vi "18_AcquisitionDataProgram.vi"() -> ()   [LabVIEW 2015]
uses:
  <vilib>/Analysis/4window.llb/windowTd.ctl
  <vilib>/DAQmx/configure/timing.llb/DAQmx Timing (Sample Clock).vi
  <vilib>/DAQmx/miscellaneous.llb/DAQmx Fill In Error Info.vi
  <vilib>/measure/maspectr.llb/FFT Power Spectrum and PSD for 1 Chan.vi
  <vilib>/DAQmx/create/channels.llb/DAQmx Create Channel (AO-Voltage-Basic).vi
  <vilib>/DAQmx/create/channels.llb/DAQmx Create Channel (AI-Voltage-Basic).vi
  <vilib>/DAQmx/read.llb/DAQmx Read (Analog Wfm 1Chan NSamp).vi
  <vilib>/measure/matone.llb/Extract Single Tone Information 1 Chan.vi
  <vilib>/DAQmx/write.llb/DAQmx Write (Analog Wfm 1Chan NSamp).vi
  <vilib>/Utility/file.llb/Write Delimited Spreadsheet (string).vi
  <vilib>/measure/NI_MABase.lvlib
  <vilib>/measure/NI_MAPro.lvlib
  <vilib>/Analysis/NI_AALPro.lvlib
panel:
  in  "Tab Control":enum32{"Page 1", "Page 2"}(tab)
  out "Waveform Graph 3":cluster{"f0":dbl, "df":dbl, "magnitude":dbl[]}(graph)
  out "Waveform Graph 2":waveform(dbl)(graph)
  out "detected frequency":dbl format="%.2p"
  out "Boolean":bool
  out "Boolean 2":bool
  out "Boolean 3":bool
  out "Boolean 4":bool
  out "Boolean 5":bool
  out "Boolean 6":bool
  in  "Save Button":bool
  in  "file path (dialog if empty)":path=path "C:/Users/student/Desktop/GrellaMarsellaOliva/configuration_tree.txt.txt"
  in  "physical channels 2":tag="Dev1/ai2"
  in  "window":T1=1 items=["Rectangle"=0, "Hanning"=1, "Hamming"=2, "Blackman-Harris"=3, "Exact Blackman"=4, "Blackman"=5, "Flat Top"=6, "4 Term B-Harris "=7, "7 Term B-Harris"=8, "Low Sidelobe"=9, "Blackman Nuttall"=11, "Triangle"=30, "Bartlett-Hanning"=31, "Bohman"=32, "Parzen"=33, "Welch"=34, "Kaiser"=60, "Dolph-Chebyshev"=61, "Gaussian"=62]
  in  "dB On":bool
  out "detected amplitude":dbl format="%.2p"
  out "Waveform Graph":waveform(dbl)(graph)
  in  "rate":string(combo)="20"
  in  "physical channels":tag="Dev1/ao0"
  in  "amplitude":dbl(knob)=2.0 scale=0.0..5.0
  in  "stop":bool
  # "Luca Grellla, Daniele Marsella, Gianluigi Oliva"
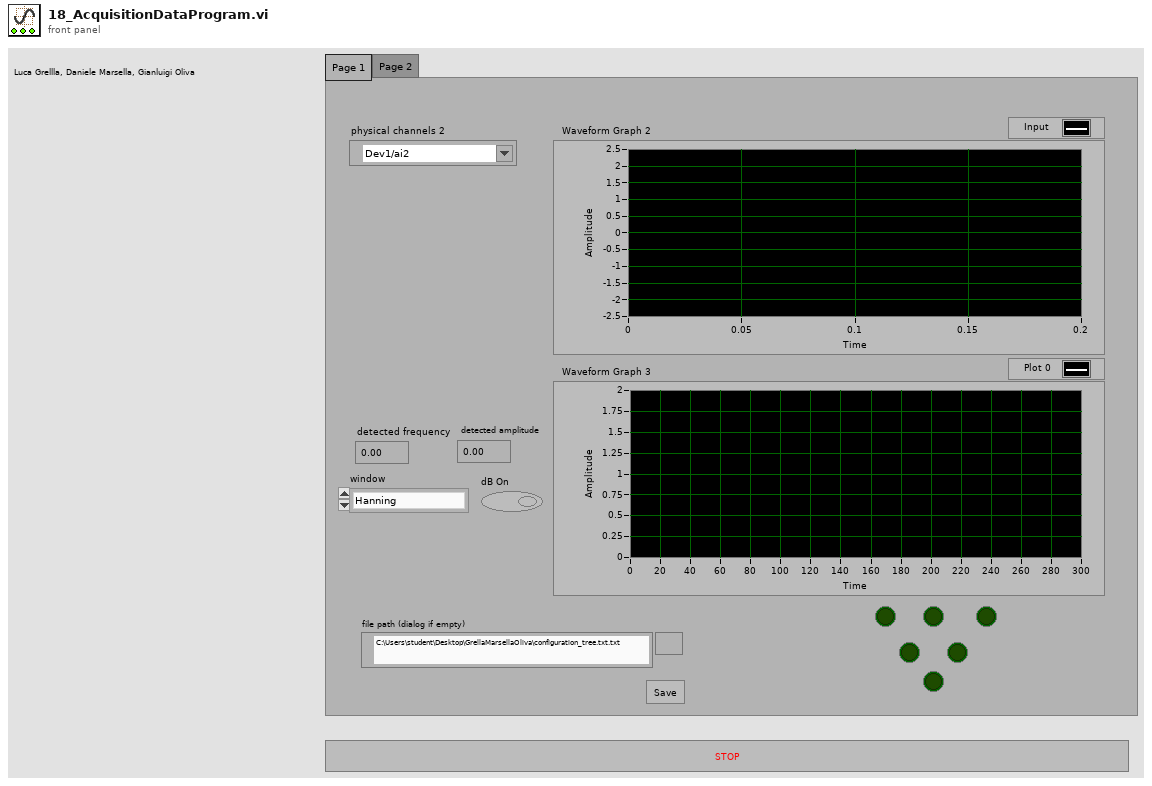
[diagram p1: front panel]
types:
  T1 = typedef "NI_AALPro.lvlib/windowTd.ctl" = u32
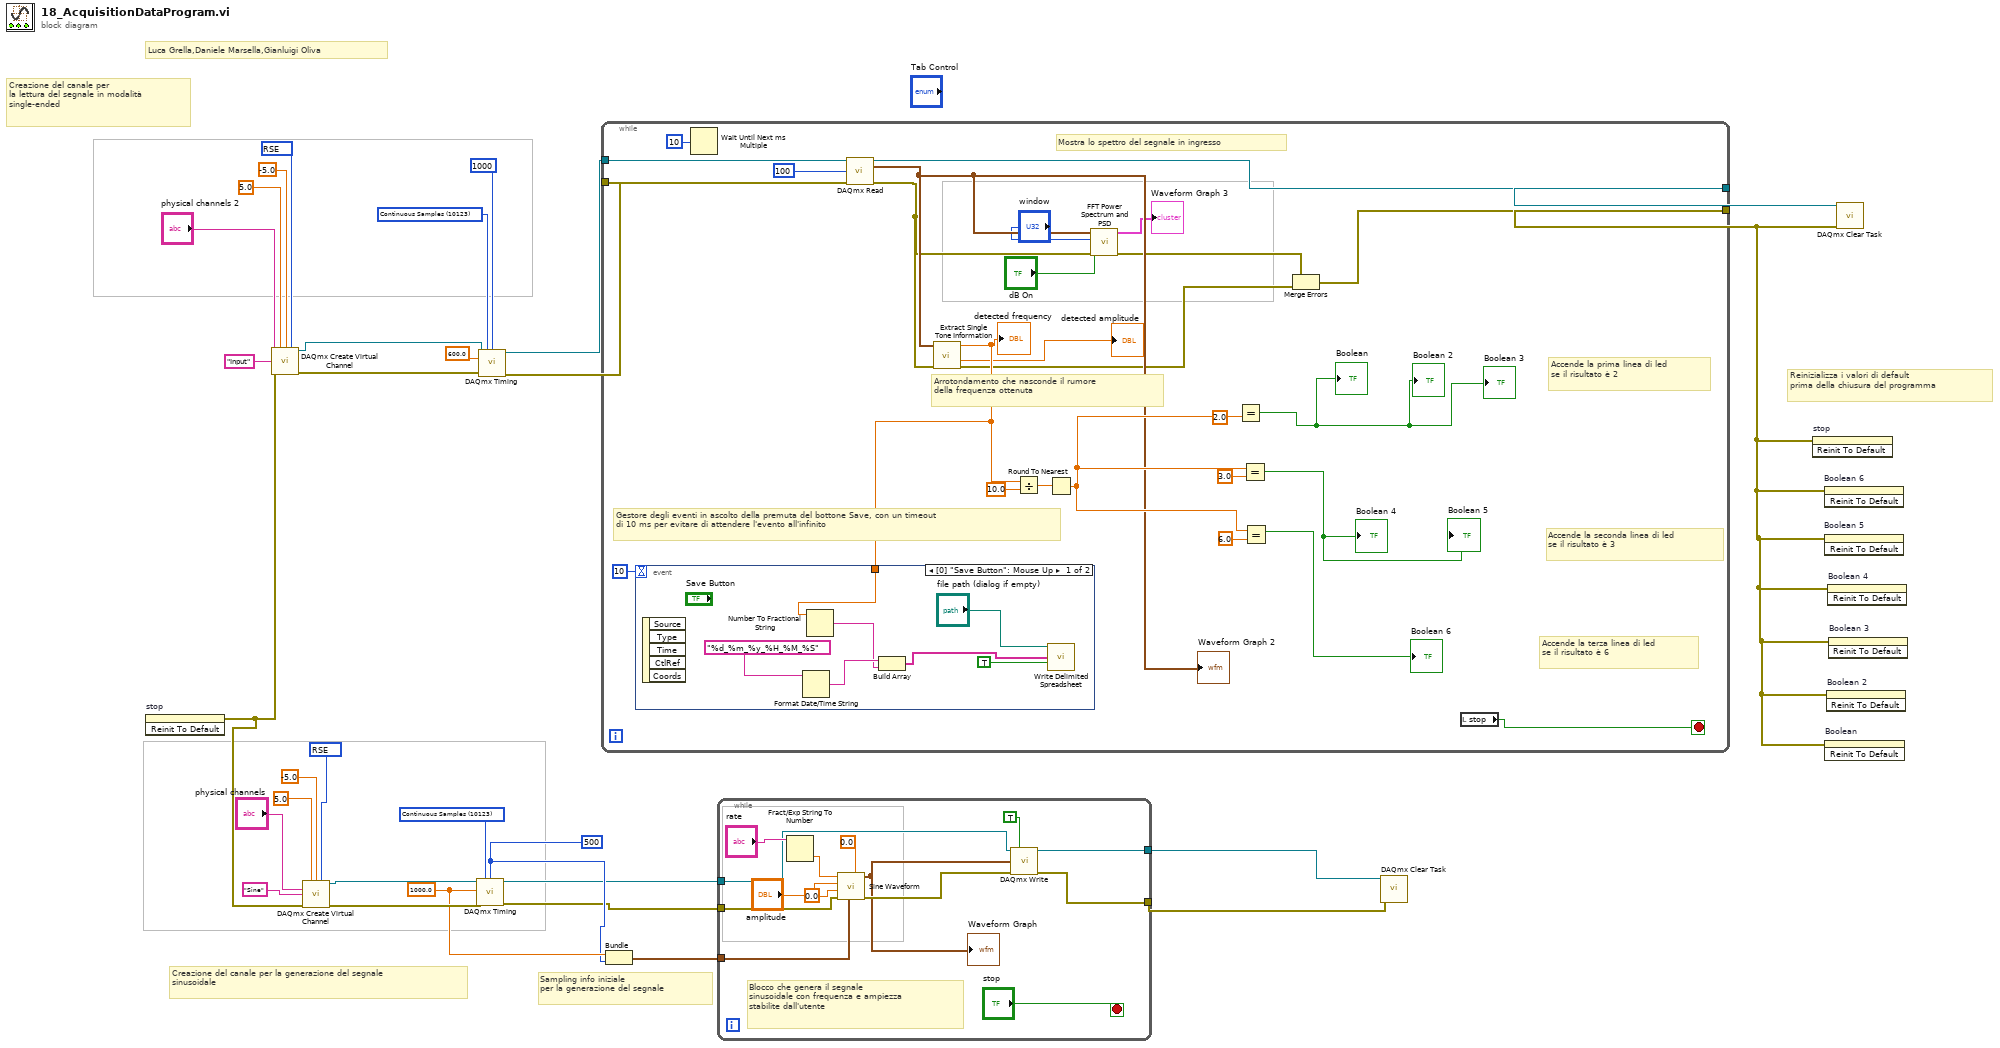
[diagram p0: block diagram]
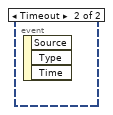
[diagram p2: hidden frame]
diagram:
  w3 = 10083 items=["Default"=-1, "RSE"=10083, "NRSE"=10078, "Differential"=10106, "Pseudodifferential"=12529] ("input terminal configuration")
  w12 = 10123 items=["Finite Samples"=10178, "Continuous Samples"=10123, "Hardware Timed Single Point"=12522] ("sample mode")
  w21 = 500 ("samples per channel")
  w22 = 1000.0 ("rate")
  w24 = 10123 items=["Finite Samples"=10178, "Continuous Samples"=10123, "Hardware Timed Single Point"=12522] ("sample mode")
  w27 = 10083 items=["Default"=-1, "RSE"=10083, "Differential"=10106, "Pseudodifferential"=12529] ("output terminal configuration")
  # "Reinizializza i valori di default\nprima della chiusura del programma"
  # "Sampling info iniziale\nper la generazione del segnale"
  # "Creazione del canale per la generazione del segnale \nsinusoidale"
  # "Creazione del canale per\nla lettura del segnale in modalità\nsingle-ended"
  # "Luca Grella,Daniele Marsella,Gianluigi Oliva"
  n1 = invoke on="stop" class="Bool (strict)" method="Reinit To Default"() -> (error out=w6:errorcluster)  [unwired: 3 in, 2 out]
  n2 = call-poly <vilib>:"DAQmx Create Virtual Channel.vi"("maximum value"=5.0, "minimum value"=-5.0, "input terminal configuration"=w3, "physical channels"="physical channels 2", "name to assign"="Input", "error in"=w6) -> ("task out"=w11:refnum<k21>, "error out"=w10:errorcluster)  [unwired: 8 in]
  n3 = call-poly <vilib>:"DAQmx Create Virtual Channel.vi"("maximum value"=5.0, "minimum value"=-5.0, "output terminal configuration"=w27, "physical channels"="physical channels", "name to assign"="Sine", "error in"=w6) -> ("task out"=w25:refnum<k21>, "error out"=w23:errorcluster)  [unwired: 8 in]
  n4 = call-poly <vilib>:"DAQmx Timing.vi"("task/channels in"=w25, "sample mode"=w24, "samples per channel"=w21, "rate"=w22, "error in"=w23) -> ("task out"=w19:refnum<k21>, "error out"=w18:errorcluster)  [unwired: 9 in]
  n5 = call-poly <vilib>:"DAQmx Timing.vi"("task/channels in"=w11, "sample mode"=w12, "samples per channel"=1000, "rate"=600.0, "error in"=w10) -> ("task out"=w8:refnum<k21>, "error out"=w7:errorcluster)  [unwired: 9 in]
  n6 = while {
    tunnel: w8 -> [w56]
    tunnel: w7 -> [w55]
    tunnel: [w53] -> w2
    tunnel: [w33] -> w1
    stop <- w54 stop-if-true
    # "Mostra lo spettro del segnale in ingresso"
    # "Accende la terza linea di led\nse il risultato è 6"
    # "Accende la seconda linea di led\nse il risultato è 3"
    # "Accende la prima linea di led\nse il risultato è 2"
    # "Arrotondamento che nasconde il rumore\ndella frequenza ottenuta"
    # "Gestore degli eventi in ascolto della premuta del bottone Save, con un timeout\ndi 10 ms per evitare di attendere l'evento all'infinito"
    n7 = Wait Until Next ms Multiple(millisecond multiple=u32 10) -> ()  [unwired: 1 out]
    n8 = call-poly <vilib>:"DAQmx Read.vi"("task/channels in"=w56, "number of samples per channel"=100 ("samples per channel"), "error in"=w55) -> ("task out"=w53:refnum<k21>, "data"=w39:waveform(dbl), "error out"=w36:errorcluster)  [unwired: 10 in]
    "Waveform Graph 2" <- w39
    n9 = call-poly <vilib>:"Extract Single Tone Information.vi"("error in (no error)"=w36, "time signal in"=w39) -> ("error out"=w35:errorcluster, "detected amplitude"=→"detected amplitude":dbl, "detected frequency"=w49:dbl)  [unwired: 4 in, 3 out]
    "detected frequency" <- w49
    n10 = event shown="[0] \"Save Button\": Mouse Up" {
      selector: _ -> [_ _]
      dyn-events: _ -> [_ _]
      timeout: 10 -> [_ _]
      tunnel: w49 -> [w59 _]
      event "Save Button": Mouse Up {
        n11 = event-data() -> ()  [unwired: 1 in, 5 out]
        n12 = Format Date/Time String(time format string (%c)="%d_%m_%y_%H_%M_%S") -> (date/time string=w62:string)  [unwired: 2 in]
        n13 = Number To Fractional String(number=w59) -> (F-format string=w58:string)  [unwired: 3 in]
        n14 = Build Array(w62, w58) -> (w57:string[])
        n15 = call-poly <vilib>:"Write Delimited Spreadsheet.vi"("file path (dialog if empty)"="file path (dialog if empty)", "1D data"=w57, "append to file? (F)"=TRUE) -> ()  [unwired: 11 in, 2 out]
      }
      event Timeout {
        n16 = event-data() -> ()  [unwired: 1 in, 3 out]
      }
    }
    n17 = Divide(x=w49, y=10.0) -> (x/y=w47:dbl)
    n18 = Round To Nearest(number=w47) -> (nearest integer value=w46:dbl)
    n19 = call-poly <vilib>:"FFT Power Spectrum and PSD.vi"("error in (no error)"=w36, "dB On (F)"="dB On", "window"="window", "time signal"=w39) -> ("error out"=w34:errorcluster, "Power Spectrum / PSD"=→"Waveform Graph 3":cluster{"f0":dbl, "df":dbl, "magnitude":dbl[]})  [unwired: 4 in, 2 out]
    n20 = Equal?(x=w46, y=2.0) -> (x = y?=→"Boolean" →"Boolean 2" →"Boolean 3":bool)
    n21 = Equal?(x=w46, y=3.0) -> (x = y?=→"Boolean 4" →"Boolean 5":bool)
    n22 = Equal?(x=w46, y=6.0) -> (x = y?=→"Boolean 6":bool)
    n23 = Merge Errors(w34, w35) -> (w33:errorcluster)
    n24 = local read "stop"() -> (w54:bool)
  }
  n25 = Bundle("rate"=w22, "samples per channel"=w21) -> (w20:cluster{"rate":dbl, "samples per channel":i32})  [unwired: 1 in]
  n26 = while {
    tunnel: w20 -> [w72]
    tunnel: w19 -> [w71]
    tunnel: w18 -> [w66]
    tunnel: [w70] -> w17
    tunnel: [w69] -> w16
    stop <- "stop" stop-if-true
    # "Blocco che genera il segnale \nsinusoidale con frequenza e ampiezza\nstabilite dall'utente"
    n27 = Fract/Exp String To Number(string="rate") -> (number=w76:dbl)  [unwired: 3 in, 1 out]
    n28 = call <vilib>:"Sine Waveform.vi"("offset"=0.0, "sampling info"=w72, "error in (no error)"=w66, "phase"=0.0, "amplitude"="amplitude", "frequency"=w76) -> ("error out"=w65:errorcluster, "signal out"=w64:waveform(dbl))  [unwired: 4 in]
    "Waveform Graph" <- w64
    n29 = call-poly <vilib>:"DAQmx Write.vi"("task/channels in"=w71, "auto start"=TRUE, "data"=w64, "error in"=w65) -> ("task out"=w70:refnum<k21>, "error out"=w69:errorcluster)  [unwired: 9 in, 1 out]
  }
  n30 = call <vilib>:"DAQmx Clear Task.vi"("task in"=w17, "error in"=w16) -> ()  [unwired: 13 in, 1 out]
  n31 = invoke on="stop" class="Bool (strict)" method="Reinit To Default"(error in=w1) -> ()  [unwired: 2 in, 3 out]
  n32 = invoke on="Boolean 6" class="Bool (strict)" method="Reinit To Default"(error in=w1) -> ()  [unwired: 2 in, 3 out]
  n33 = invoke on="Boolean 5" class="Bool (strict)" method="Reinit To Default"(error in=w1) -> ()  [unwired: 2 in, 3 out]
  n34 = invoke on="Boolean" class="Bool (strict)" method="Reinit To Default"(error in=w1) -> ()  [unwired: 2 in, 3 out]
  n35 = invoke on="Boolean 2" class="Bool (strict)" method="Reinit To Default"(error in=w1) -> ()  [unwired: 2 in, 3 out]
  n36 = invoke on="Boolean 4" class="Bool (strict)" method="Reinit To Default"(error in=w1) -> ()  [unwired: 2 in, 3 out]
  n37 = invoke on="Boolean 3" class="Bool (strict)" method="Reinit To Default"(error in=w1) -> ()  [unwired: 2 in, 3 out]
  n38 = call <vilib>:"DAQmx Clear Task.vi"("task in"=w2, "error in"=w1) -> ()  [unwired: 13 in, 1 out]
